vi "PDF Protokoll EPA1065_550 Drift.vi"(8 "error in (no error)":errorcluster caption="Fehler (Eingang, kein Fehler)") -> (0 "error out":errorcluster caption="Fehler (Ausgang)")   [LabVIEW 2020, in "EPA 1065.lvlib" / "Gas Analyzer Drift 1065-550.lvlib"]
uses:
  Gas Analyzer Drift 1065-550.lvlib
  Drifttabelle.ctl
  Seiten/FT-IR/FGV FT-IR Aktionen.ctl
  Chiller NO2 1065-376/Aktion FGV Drift Daten.ctl
  Seiten/System Einstellungen V2/Aktioen FGV System Konstanten.ctl
  <vilib>/Utility/miscctls.llb/LVPrintingMarginsTypeDef.ctl
  Allgemein/allgemeine Sub-VIs.lvlib
  Seiten/FT-IR/FT-IR.lvlib
  Seiten/System Einstellungen V2/System Einstellungen V2.lvlib
panel:
  out "Drifttabelle":T1
  out "Versa Serial number:":string caption="Serial number:"
  out "Anlage:":string caption="Measuring Device:"
  out "Methode (Recipe):":string
  out "Date & Time:":string
  out "Bearbeiter:":string caption="Operator:"
  # "Drift Test EPA § 1065.550"
  # "x"
  # "x"
  # "x"
  # "x"
  # "x"
  # "x"
  # "xidriftcorrected=xrefzero+(xrefspan-xrefzero)·2xi-(xprezero+xpostzero)(xprespan+xpostspan)-(xprezero+xpostzero)"
  # "Eq. 1065.672-1"
  # "xidriftcorrected = concentration corrected for drift."
  # "xrefzero = reference concentration of the zero gas, which is usually zero unless known to be otherwise."
  # "xrefspan = reference concentration of the span gas."
  # "xprespan = pre-test interval gas analyzer response to the span gas concentration."
  # "xpostspan = post-test interval gas analyzer response to the span gas concentration."
  # "xi or x = concentration recorded during test, before drift correction."
  # "xprezero = pre-test interval gas analyzer response to the zero gas concentration."
  # "xpostzero = post-test interval gas analyzer response to the zero gas concentration."
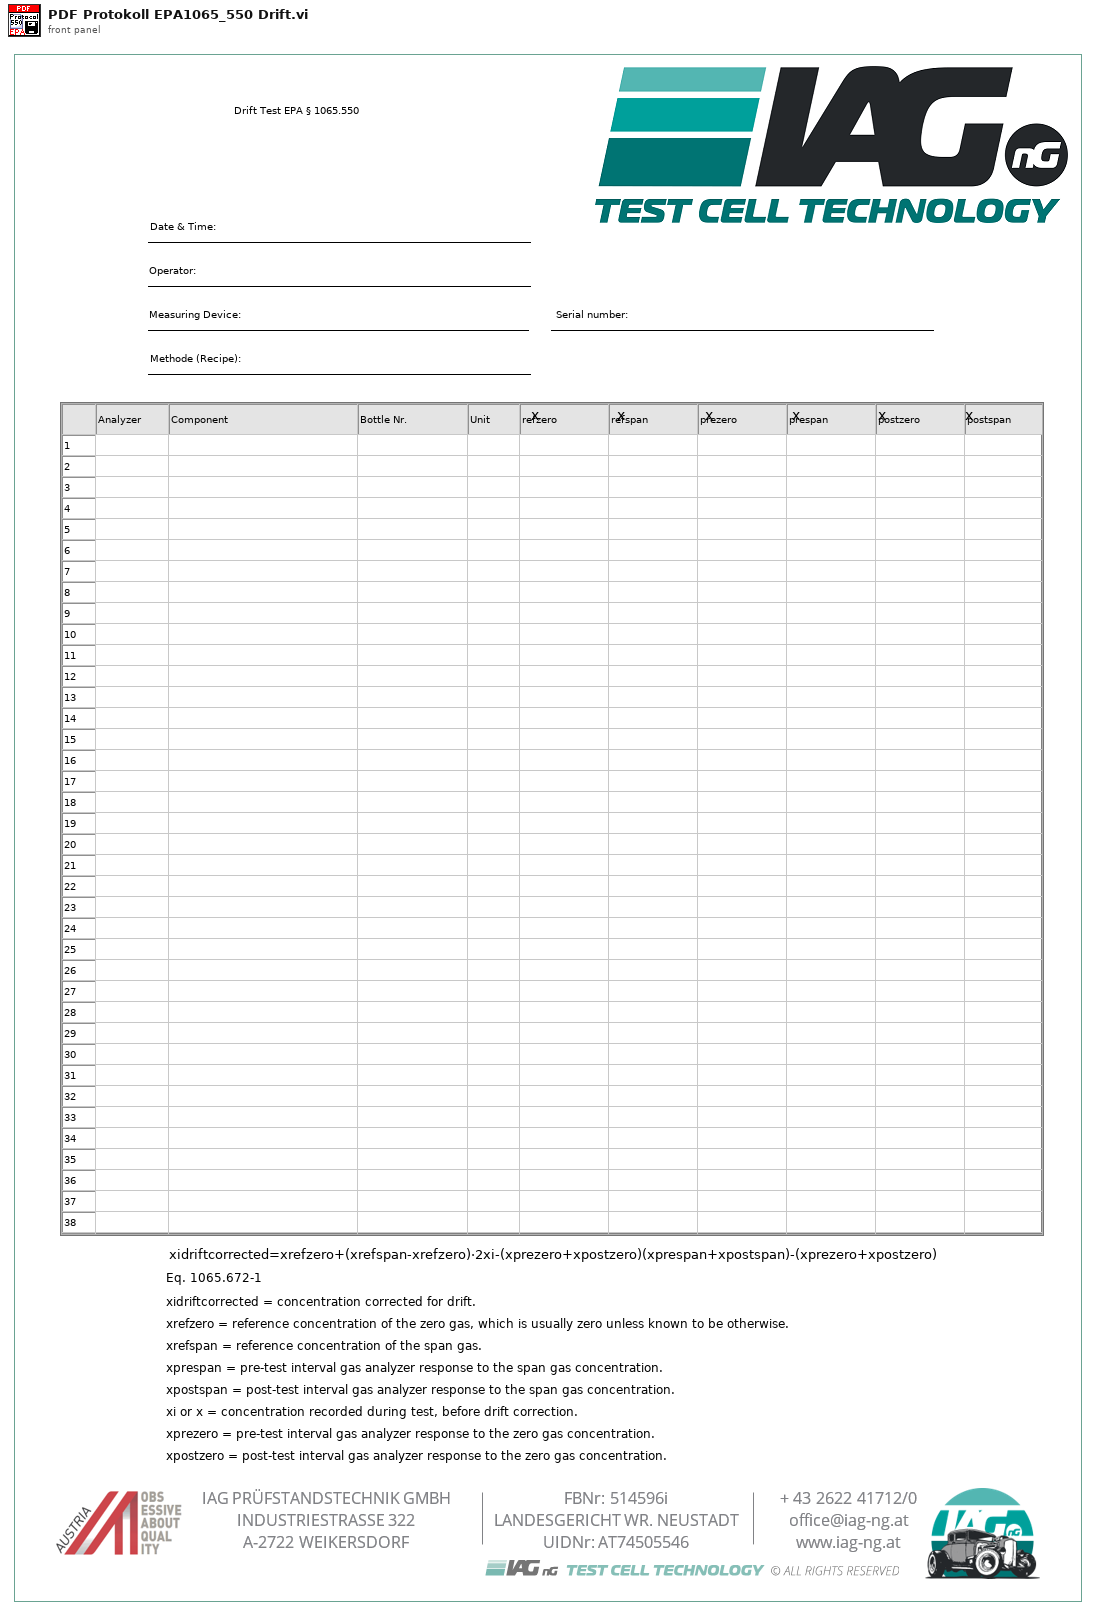
[diagram p1: front panel]
types:
  T1 = typedef "EPA 1065.lvlib/Gas Analyzer Drift 1065-550.lvlib/Drifttabelle.ctl" = string[][]
  T2 = typedef "System Einstellungen V2.lvlib/Aktioen FGV System Konstanten.ctl" = enum16{"lesen", "laden", "speichern", "Sprache"}
  T3 = typedef "EPA 1065.lvlib/Gas Analyzer Drift 1065-550.lvlib/Aktion FGV Drift Daten.ctl" = enum16{"lesen", "Konfig Daten", "PDF einstellen", "laden", "speichern", "Tabelle init", "Zeile Prüfen", "Info schreiben", "Span Einstellung", "Pre Werte schreiben", "Post Werte schreiben", "NB Pre Wert schreiben", "NB Post Wert schreiben", "Tabelle löschen"}
  T4 = typedef "FT-IR.lvlib/FGV FT-IR Aktionen.ctl" = enum16{"lesen", "NOG setzen", "NOS setzen", "Initialisieren", "speichern", "ALLES setzen", "FT-IR Spektrum loggen", "Komm Stoppen", "Spektrum LogKonfig"}
  T5 = enum32{"Portrait", "Landscape", "Rotated Portrait", "Rotated Landscape"}
  T6 = typedef "LVPrintingMarginsTypeDef.ctl" = cluster{"Top":sgl, "Left":sgl, "Bottom":sgl, "Right":sgl, "Measurement System":enum8{"Inches", "cm"}}
  T7 = typedef "EPA 1065.lvlib/Gas Analyzer Drift 1065-550.lvlib/Konfig Daten Drift Verification.ctl" = cluster{"Bearbeiter:":string, "Pfad:":path, "Textname:":string, "CG Aufschaltzeit:":dbl, "N2 Aufschaltzeit:":dbl}
  T8 = cluster{"Modell":string, "ProjektNummer":string, "Software Version":string, "Seriennummer":string}
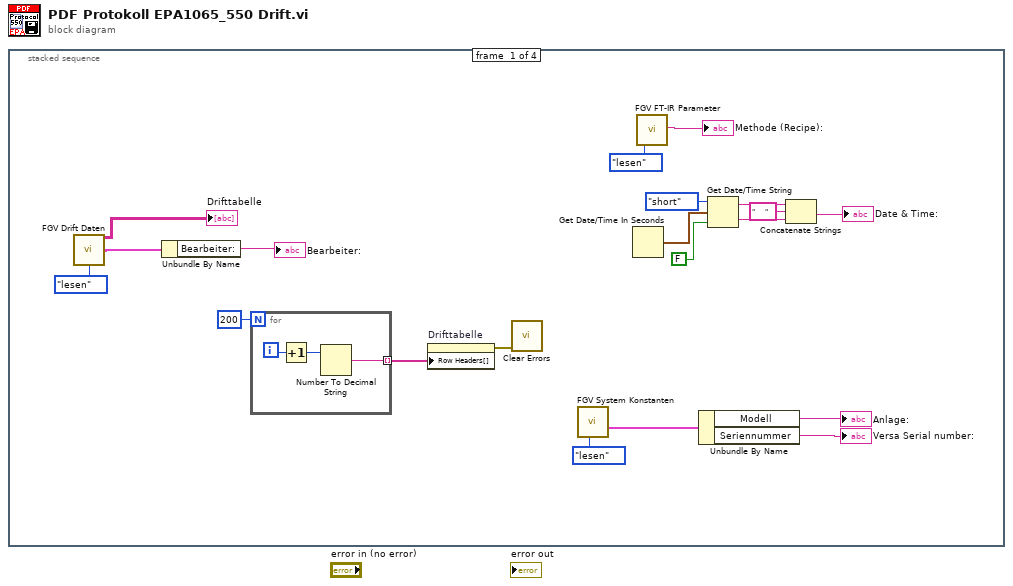
[diagram p0: block diagram]
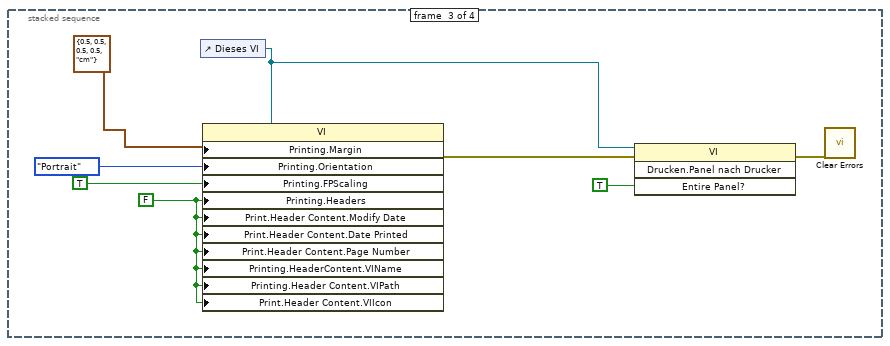
[diagram p3: hidden frame]
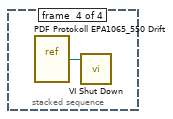
[diagram p4: hidden frame]
diagram:
  n1 = stacked-sequence {
    frame #0 {
      n2 = call "FGV Drift Daten.vi"("Aktion"=Aktion_FGV_Drift_Daten."lesen") -> ("Drifttabelle"=→"Drifttabelle":T1, "Drift Konfig Daten"=w8:T7)  [unwired: 7 in, 6 out]
      n3 = Unbundle By Name(w8) -> ("Bearbeiter:"=→"Bearbeiter:":string)
      n4 = for {
        N: 200 -> [_]
        tunnel: [w21] -> w5 mode=indexing
        i -> [w23]
        n5 = Increment(x=w23) -> (x+1=w22:i32)
        n6 = Number To Decimal String(number=w22) -> (decimal integer string=w21:string)  [unwired: 1 in]
      }
      n7 = property on="Drifttabelle" class="Tbl (strikt)"("Row Headers[]"=w5) -> (error out=w4:errorcluster)  [unwired: 2 in, 1 out]
      n8 = call <vilib>:"Clear Errors.vi"("error in (no error)"=w4) -> ()  [unwired: 5 in, 2 out]
      n9 = call "FGV System Konstanten.vi"("Aktionen"=Aktioen_FGV_System_Konstanten."lesen") -> ("Cluster out"=w2:T8)  [unwired: 6 in, 4 out]
      n10 = Get Date/Time In Seconds() -> (seconds since 1Jan1904=w20:timestamp)
      n11 = call "FGV FT-IR Parameter.vi"("Aktion"=FGV_FT-IR_Aktionen."lesen") -> ("Current Recipe"=→"Methode (Recipe):":string)  [unwired: 11 in, 7 out]
      n12 = Unbundle By Name(w2) -> ("Modell"=→"Anlage:":string, "Seriennummer"=→"Versa Serial number:":string)
      n13 = Get Date/Time String(date format (0)=enum16{"short", "long", "abbreviated"}."short" ("Datumsformat (0)"), seconds (now)=w20, want seconds? (F)=FALSE ("Angabe von Sekunden? (F)")) -> (date string=w19:string, time string=w18:string)
      n14 = Concatenate Strings(w19, "     " ("String"), w18) -> (→"Date & Time:":string)
    }
    frame #1 {
    }
    frame #2 {
      w27 = FALSE ("Drucken:Kopfzeilen?")
      n15 = control-ref of="Dieses VI"() -> (w24:refnum<vi>)
      n16 = property class="VI"(reference=w24, "Printing.Margin"=T6 {"Top"=0.5, "Left"=0.5, "Bottom"=0.5, "Right"=0.5, "Measurement System"=enum."cm"} ("Drucken:Ränder"), "Printing.Orientation"=T5."Portrait" ("Drucken:Seitenausrichtung"), "Printing.FPScaling"=TRUE ("Drucken:Frontpanel-Skalierung?"), "Printing.Headers"=w27, "Print.Header Content.Modify Date"=w27, "Print.Header Content.Date Printed"=w27, "Print.Header Content.Page Number"=w27, "Printing.HeaderContent.VIName"=w27, "Printing.Header Content.VIPath"=w27, "Print.Header Content.VIIcon"=w27) -> (error out=w31:errorcluster)  [unwired: 1 in, 1 out]
      n17 = invoke class="VI" method="Drucken.Panel nach Drucker"(reference=w24, error in=w31, "Entire Panel?"=TRUE ("Abschnittskopfzeilen?")) -> (error out=w25:errorcluster)  [unwired: 1 in, 3 out]
      n18 = call <vilib>:"Clear Errors.vi"("error in (no error)"=w25) -> ()  [unwired: 5 in, 2 out]
    }
    frame #3 {
      n19 = vi-ref "PDF Protokoll EPA1065_550 Drift.vi"() -> (w32:refnum<vi>)
      n20 = call "VI Shut Down.vi"("VI Referenz"=w32) -> ()  [unwired: 11 in]
    }
  }
